vi "GetVISAResources.vi"(8 "Error In":errorcluster) -> (0 "Error Out":errorcluster, 3 "VISA Resources":string[](array[string]))   [LabVIEW 2013, in "LV-Utilities.lvlib"]
uses:
  LV-Utilities.lvlib
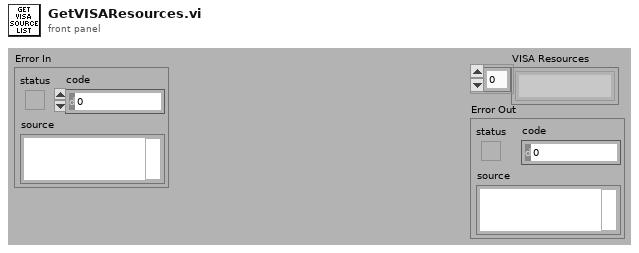
[diagram p1: front panel]
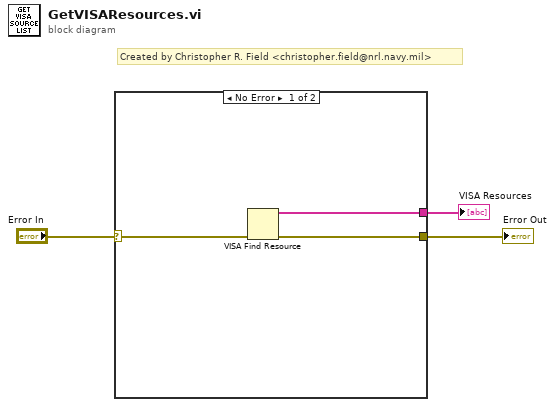
[diagram p0: block diagram]
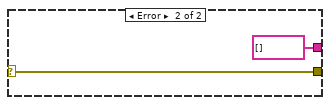
[diagram p2: hidden frame]
diagram:
  # "Created by Christopher R. Field <christopher.field@nrl.navy.mil>"
  n1 = case shown="No Error" "Error In" {
    selector: "Error In" -> [w4 w7]
    tunnel: [w6 string[] [] ("find list")] -> w3
    tunnel: [w5 w7] -> w2
    frame No Error {
      n2 = VISA Find Resource(8:w4) -> (0:w5:errorcluster, 3:w6:string[])  [unwired: 2 in, 1 out]
    }
    frame Error {
    }
  }
  "VISA Resources" <- w3
  "Error Out" <- w2
